vi "LabView_LINX_PCA9685_Servo Run.vi"() -> ()   [LabVIEW 2015]
uses:
  <vilib>/MakerHub/LINX/Private/Local IO/LinxI2cWrite.vi
  <vilib>/MakerHub/LINX/Public/Utilities/Check Channel.vi
  <vilib>/MakerHub/LINX/Public/Utilities/Open Serial.vi
  <vilib>/MakerHub/LINX/Private/Utilties/Generate Error.vi
  <vilib>/MakerHub/LINX/LMH-LINX.lvlib
panel:
  out "hi(x)":u8 format="%x"
  in  "x":u16(knob)=1000 min=1000 max=2500 step=100 scale=500.0..4000.0
  out "Error Out":errorcluster
  in  "stop":bool
  in  "Serial Port":refnum<visa-resource-name>="N/A"
  # "LED ON \nInteger value = 500"
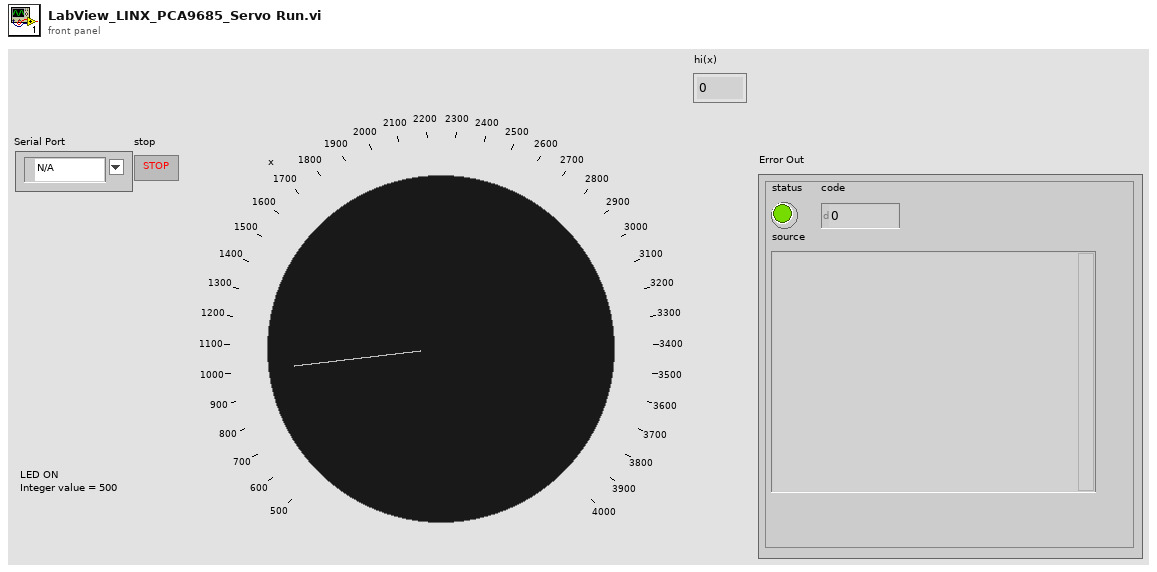
[diagram p1: front panel]
types:
  T1 = typedef "LMH-LINX.lvlib/LINX Ref.ctl" = cluster{"IO":T2, "Interface":T3, "LINX Device Config":T4}
  T2 = typedef "LMH-LINX.lvlib/Platform.ctl" = enum16{"Remote", "Local"}
  T3 = typedef "LMH-LINX.lvlib/Interface.ctl" = enum16{"Serial", "TCP"}
  T4 = typedef "LMH-LINX.lvlib/Device.lvlib/LINX Device Config.ctl" = cluster{"Interface":T3, "COM Port":refnum<visa-resource-name>, "TCP Configuration":T5, "Device Family":u8, "Device ID":u8, "Device Name":string, "TCP Ref":refnum<k5>, "Channels":T6}
  T5 = typedef "LMH-LINX.lvlib/Device.lvlib/TCP Config.ctl" = cluster{"IP Address":string, "Port":u16}
  T6 = typedef "LMH-LINX.lvlib/Channels.ctl" = cluster{"DI":u8[], "DO":u8[], "AI":u8[], "AO":u8[], "PWM":u8[], "QE":u8[], "UART":u8[], "I2C 2":u8[], "SPI":u8[], "CAN":u8[], "Servo":u8[], "AI Ref (V)":dbl, "AI Resolution (Bits)":u8, "AO Ref (V)":dbl, "AO Resolution (Bits)":u8}
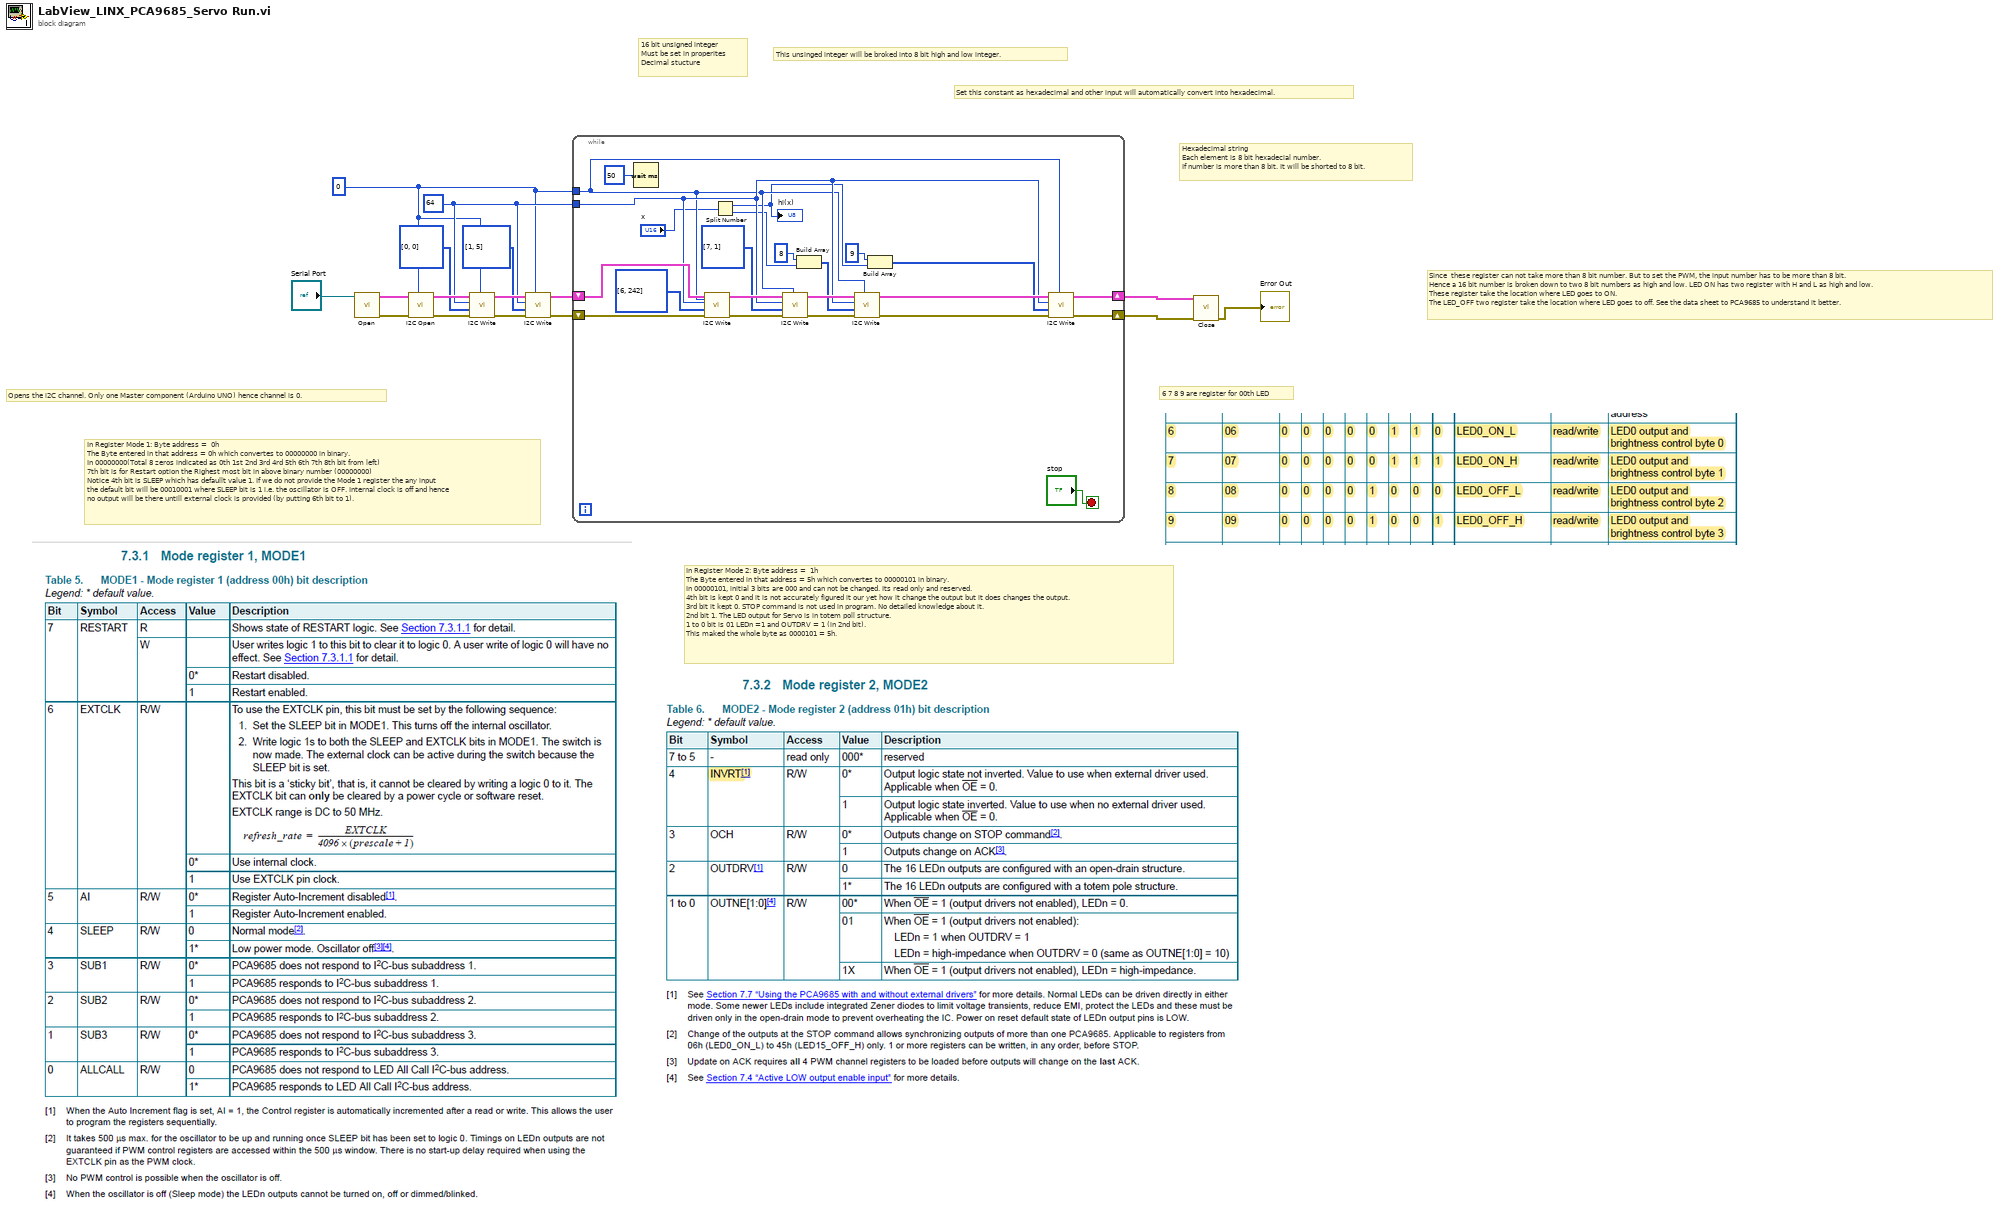
[diagram p0: block diagram]
diagram:
  w6 = u8 64
  w5 = u8 0 ("I2C Channel (0)")
  # "Since  these register can not take more than 8 bit number. But to set the PWM, the input number has to be more than 8 bit. \nHence a 16 bit number is broken down to two 8 bit numbers as high and low. LED ON has two register with H and L as high and low.\nThese register take the location where LED goes to ON. \nThe LED_OFF two register take the location where LED goes to off. See the data sheet to PCA9685 to understand it better."
  # "6 7 8 9 are register for 00th LED"
  # "Hexadecimal string\nEach element is 8 bit hexadecial number.\nIf number is more than 8 bit. It will be shorted to 8 bit."
  # "Set this constant as hexadecimal and other input will automatically convert into hexadecimal."
  # "This unsinged integer will be broked into 8 bit high and low integer."
  # "16 bit unsigned integer \nMust be set in properites\nDecimal stucture"
  # "In Register Mode 2: Byte address =  1h \nThe Byte entered in that address = 5h which convertes to 00000101 in binary. \nIn 00000101, initial 3 bits are 000 and can not be changed. Its read only and reserved.\n4th bit is kept 0 and it is not accurately figured it our yet how it change the output but it does changes the output. \n3rd bit it kept 0. STOP command is not used in program. No detailed knowledge about it. \n2nd bit 1. The LED output for Servo is in totem poll structure. \n1 to 0 bit is 01 LEDn =1 and OUTDRV = 1 (in 2nd bit).\nThis maked the whole byte as 0000101 = 5h."
  # "Opens the i2C channel. Only one Master component (Arduino UNO) hence channel is 0."
  # "In Register Mode 1: Byte address =  0h \nThe Byte entered in that address = 0h which convertes to 00000000 in binary. \nIn 00000000(Total 8 zeros indicated as 0th 1st 2nd 3rd 4rd 5th 6th 7th 8th bit from left)\n7th bit is for Restart option the Righest most bit in above binary number (00000000)\nNotice 4th bit is SLEEP which has defaullt value 1. If we do not provide the Mode 1 register the any input \nthe default bit will be 00010001 where SLEEP bit is 1 i.e. the oscillator is OFF. Internal clock is off and hence \nno output will be there untill external clock is provided (by putting 6th bit to 1)."
  n1 = call-poly <vilib>:"Open.vi"("Serial Port"="Serial Port") -> ("Error Out"=w11:errorcluster, "LINX Resource"=w12:T1)  [unwired: 8 in, 1 out]
  n2 = call <vilib>:"I2C Open.vi"("I2C Channel (0)"=w5, "Error In"=w11, "LINX Resource"=w12) -> ("Error Out"=w1:errorcluster, "LINX Resource"=w10:T1)  [unwired: 7 in]
  n3 = call <vilib>:"I2C Write.vi"("I2C Channel"=w5, "Error In"=w1, "Data"=u8[] [0, 0], "I2C Slave Address (0)"=w6, "LINX Resource"=w10) -> ("Error Out"=w2:errorcluster, "LINX Resource"=w9:T1)  [unwired: 5 in]
  n4 = call <vilib>:"I2C Write.vi"("I2C Channel"=w5, "Error In"=w2, "Data"=u8[] [1, 5], "I2C Slave Address (0)"=w6, "LINX Resource"=w9) -> ("Error Out"=w3:errorcluster, "LINX Resource"=w7:T1)  [unwired: 5 in]
  n5 = while {
    shift-right: [w31] -> w15
    shift-left: w7 -> [w38]
    shift-right: [w30] -> w14
    shift-left: w3 -> [w37]
    tunnel: w5 -> [w25]
    tunnel: w6 -> [w26]
    stop <- "stop" stop-if-true
    n6 = Wait (ms)(milliseconds to wait=u32 50) -> ()  [unwired: 1 out]
    n7 = call <vilib>:"I2C Write.vi"("I2C Channel"=w25, "Error In"=w37, "Data"=u8[] [6, 242], "I2C Slave Address (0)"=w26, "LINX Resource"=w38) -> ("Error Out"=w27:errorcluster, "LINX Resource"=w35:T1)  [unwired: 5 in]
    n8 = Split Number(x="x") -> (hi(x)=w21:u8, lo(x)=w20:u8)
    "hi(x)" <- w21
    n9 = call <vilib>:"I2C Write.vi"("I2C Channel"=w25, "Error In"=w27, "Data"=u8[] [7, 1], "I2C Slave Address (0)"=w26, "LINX Resource"=w35) -> ("Error Out"=w28:errorcluster, "LINX Resource"=w34:T1)  [unwired: 5 in]
    n10 = Build Array(8, w20) -> (w17:i32[])
    n11 = call <vilib>:"I2C Write.vi"("I2C Channel"=w25, "Error In"=w28, "Data"=w17, "I2C Slave Address (0)"=w26, "LINX Resource"=w34) -> ("Error Out"=w29:errorcluster, "LINX Resource"=w33:T1)  [unwired: 5 in]
    n12 = Build Array(9, w21) -> (w18:i32[])
    n13 = call <vilib>:"I2C Write.vi"("I2C Channel"=w25, "Error In"=w29, "Data"=w18, "I2C Slave Address (0)"=w26, "LINX Resource"=w33) -> ("Error Out"=w30:errorcluster, "LINX Resource"=w31:T1)  [unwired: 5 in]
  }
  n14 = call <vilib>:"Close.vi"("Error In"=w14, "LINX Resource"=w15) -> ("Error Out"=→"Error Out":errorcluster)  [unwired: 9 in]
